vi "OCV Stream Asynchronous.vi"(9 "Physical Channel":tag, 10 "Rate (Hz)":dbl, 11 "gRPCid":T1) -> (0 "error out":errorcluster)   [LabVIEW 2019]
uses:
  labview-grpc-query-server/VIs/MeasurementServer_gRPCid.ctl
  Global Operations.ctl
  labview-grpc-query-server/VIs/MeasurementServer_ErrorOutData.ctl
  labview-grpc-query-server/VIs/MeasurementServer_OCVRawData.ctl
  labview-grpc-query-server/VIs/labview-grpc-measurement-server.lvlib
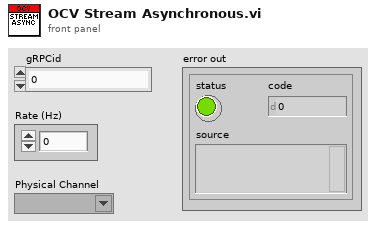
[diagram p1: front panel]
types:
  T1 = typedef "labview-grpc-measurement-server.lvlib/MeasurementServer_gRPCid.ctl" = u64
  T2 = typedef "Global Operations.ctl" = enum16{"Get", "Set"}
  T3 = typedef "labview-grpc-measurement-server.lvlib/MeasurementServer_OCVRawData.ctl" = cluster{"battery1voltage":sgl, "battery2voltage":sgl, "battery3voltage":sgl, "battery4voltage":sgl, "battery5voltage":sgl, "battery6voltage":sgl, "battery7voltage":sgl, "battery8voltage":sgl, "battery9voltage":sgl, "battery10voltage":sgl, "battery11voltage":sgl, "battery12voltage":sgl, "battery13voltage":sgl, "battery14voltage":sgl, "battery15voltage":sgl, "battery16voltage":sgl, "battery17voltage":sgl, "battery18voltage":sgl, "battery19voltage":sgl, "battery20voltage":sgl, "battery21voltage":sgl, "battery22voltage":sgl, "battery23voltage":sgl, "battery24voltage":sgl, "ErrorOutData":T4}
  T4 = typedef "labview-grpc-measurement-server.lvlib/MeasurementServer_ErrorOutData.ctl" = cluster{"ErrorCode":i32, "ErrorMessage":string}
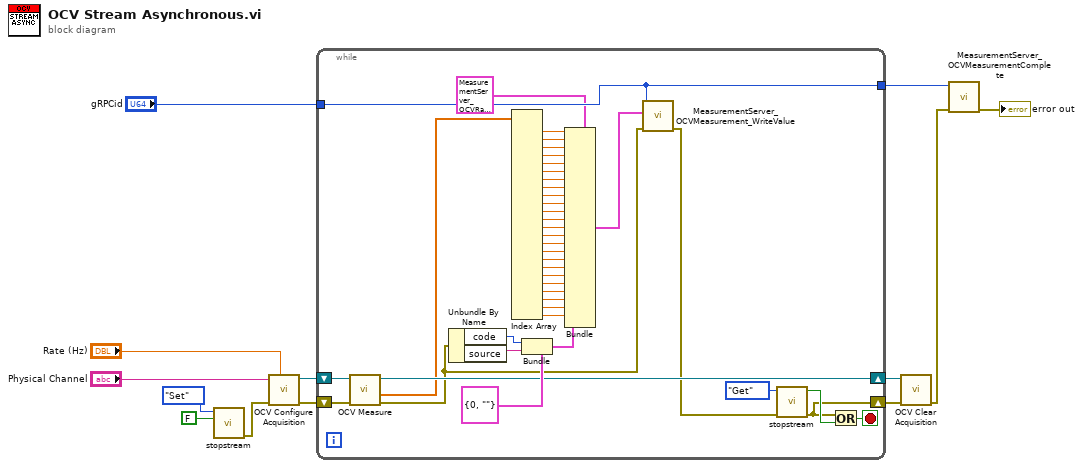
[diagram p0: block diagram]
diagram:
  n1 = call "stopstream.vi"("STOPSTREAM"=FALSE, "Operation"=Global_Operations."Set") -> ("error out"=w13:errorcluster)  [unwired: 8 in, 1 out]
  n2 = call "OCV Configure Acquisition.vi"("Rate (Hz)"="Rate (Hz)", "error in (no error)"=w13, "Physical Channel"="Physical Channel") -> ("error out"=w6:errorcluster, "Refnum out"=w5:refnum<k21>)  [unwired: 6 in, 1 out]
  n3 = while {
    tunnel: "gRPCid" -> [w54]
    tunnel: [w54] -> w2
    shift-right: [w42] -> w3
    shift-left: w5 -> [w40]
    shift-right: [w36] -> w4
    shift-left: w6 -> [w39]
    stop <- w37 stop-if-true
    n4 = call "OCV Measure.vi"("error in (no error)"=w39, "Refnum in"=w40) -> ("error out"=w34:errorcluster, "Voltage"=w41:sgl[], "Refnum out"=w42:refnum<k21>)  [unwired: 6 in, 1 out]
    n5 = Unbundle By Name(w34) -> ("code"=w52:i32, "source"=w51:string)
    n6 = Index Array(array=w41) -> (element #1=w49:sgl, element #2=w48:sgl, element #3=w47:sgl, element #4=w46:sgl, element #5=w45:sgl, element #6=w32:sgl, element #7=w31:sgl, element #8=w30:sgl, element #9=w29:sgl, element #10=w28:sgl, element #11=w27:sgl, element #12=w26:sgl, element #13=w25:sgl, element #14=w23:sgl, element #15=w24:sgl, element #16=w22:sgl, element #17=w21:sgl, element #18=w20:sgl, element #19=w19:sgl, element #20=w18:sgl, element #21=w17:sgl, element #22=w16:sgl, element #23=w15:sgl, element #24=w14:sgl)  [unwired: 24 in]
    n7 = Bundle(cluster=T4 {"ErrorCode"=0, "ErrorMessage"=""} ("ErrorOutData"), "ErrorCode"=w52, "ErrorMessage"=w51) -> (w50:T4)
    n8 = Bundle(cluster=T3 {"battery1voltage"=0.0, "battery2voltage"=0.0, "battery3voltage"=0.0, "battery4voltage"=0.0, "battery5voltage"=0.0, "battery6voltage"=0.0, "battery7voltage"=0.0, "battery8voltage"=0.0, "battery9voltage"=0.0, "battery10voltage"=0.0, "battery11voltage"=0.0, "battery12voltage"=0.0, "battery13voltage"=0.0, "battery14voltage"=0.0, "battery15voltage"=0.0, "battery16voltage"=0.0, "battery17voltage"=0.0, "battery18voltage"=0.0, "battery19voltage"=0.0, "battery20voltage"=0.0, "battery21voltage"=0.0, "battery22voltage"=0.0, "battery23voltage"=0.0, "battery24voltage"=0.0, "ErrorOutData"={"ErrorCode"=0, "ErrorMessage"=""}} ("OCVRawData"), "battery1voltage"=w49, "battery2voltage"=w48, "battery3voltage"=w47, "battery4voltage"=w46, "battery5voltage"=w45, "battery6voltage"=w32, "battery7voltage"=w31, "battery8voltage"=w30, "battery9voltage"=w29, "battery10voltage"=w28, "battery11voltage"=w27, "battery12voltage"=w26, "battery13voltage"=w25, "battery14voltage"=w23, "battery15voltage"=w24, "battery16voltage"=w22, "battery17voltage"=w21, "battery18voltage"=w20, "battery19voltage"=w19, "battery20voltage"=w18, "battery21voltage"=w17, "battery22voltage"=w16, "battery23voltage"=w15, "battery24voltage"=w14, "ErrorOutData"=w50) -> (w43:T3)
    n9 = call "MeasurementServer_OCVMeasurement_WriteValue.vi"("gRPCid"=w54, "OCVRawData"=w43, "error in (no error)"=w34) -> ("error out"=w33:errorcluster)  [unwired: 7 in]
    n10 = call "stopstream.vi"("error in (no error)"=w33, "Operation"=Global_Operations."Get") -> ("error out"=w36:errorcluster, "STOPSTREAM?"=w38:bool)  [unwired: 8 in]
    n11 = Or(x=w36, y=w38) -> (x .or. y?=w37:bool)
  }
  n12 = call "OCV Clear Acquisition.vi"("error in (no error)"=w4, "Refnum in"=w3) -> ("error out"=w9:errorcluster)  [unwired: 8 in, 1 out]
  n13 = call "MeasurementServer_OCVMeasurementComplete.vi"("gRPCid"=w2, "error in (no error)"=w9) -> ("error out"=→"error out":errorcluster)  [unwired: 8 in]
